vi "File Exists.vi"(8 "error in":errorcluster, 11 "File Path":path) -> (0 "error out":errorcluster, 2 "Exists":bool, 3 "File Path (dup)":path)   [LabVIEW 2024, in "Common Helpers.lvlib"]
uses:
  Common Helpers.lvlib
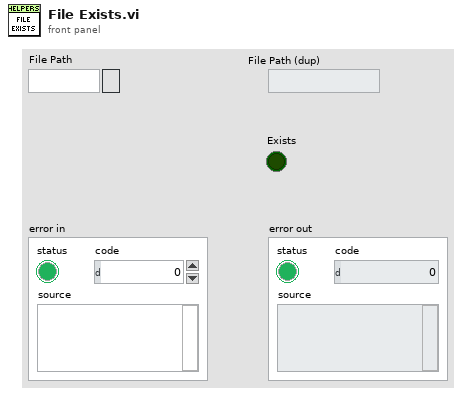
[diagram p1: front panel]
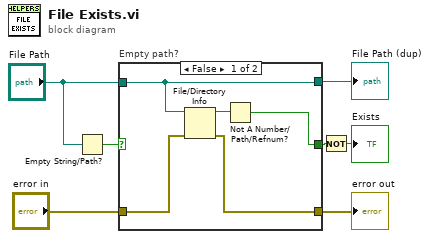
[diagram p0: block diagram]
diagram:
  n1 = Empty String/Path?(string/path="File Path") -> (empty?=w5:bool)
  n2 = case "Empty path?" shown="False" w5 {
    selector: w5 -> [_ w15]
    tunnel: "File Path" -> [w10 w14]
    tunnel: [w12 w13] -> w7
    tunnel: [w10 w14] -> w6
    tunnel: "error in" -> [w11 w13]
    tunnel: [w8 w15] -> w2
    frame False {
      n3 = File/Directory Info(path=w10, error in=w11) -> (path out=w9:path, error out=w12:errorcluster)  [unwired: 5 out]
      n4 = Not A Number/Path/Refnum?(number/path/refnum=w9) -> (NaN/Path/Refnum?=w8:bool)
    }
    frame True {
    }
  }
  "error out" <- w7
  "File Path (dup)" <- w6
  n5 = Not(x=w2) -> (.not. x?=→"Exists":bool)
